vi "sub_DL950_global-settings.vi"(11 "TestType":T1) -> (3 "String":string)   [LabVIEW 2019]
uses:
  Durability/sequence_single.ctl
  _ctrl/rw.ctl
  SubVIs/common/Glob_Ref.vi
  Durability/common/Global 1.vi
panel:
  out "String 2":string
  out "array":string[](array[string])
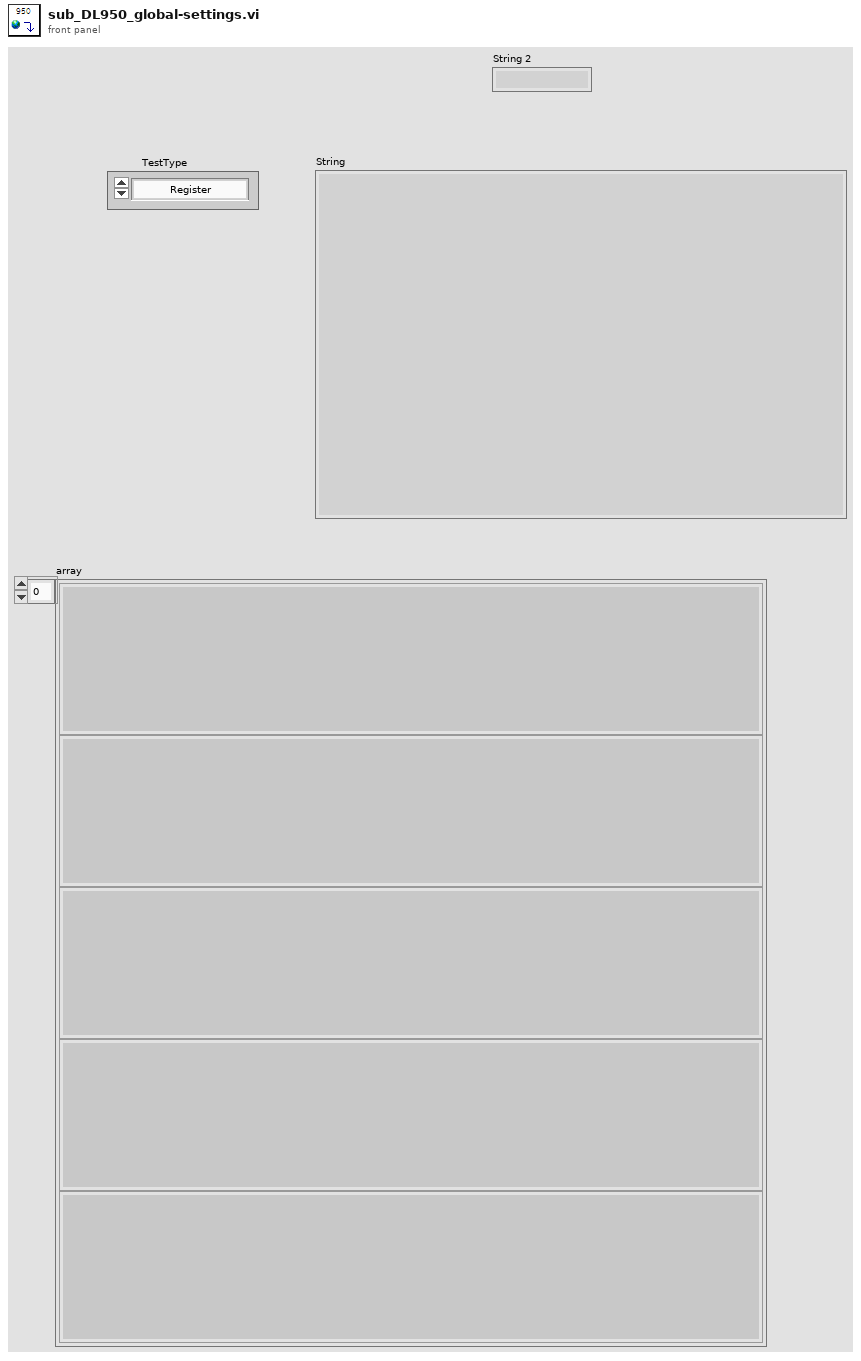
[diagram p1: front panel]
types:
  T1 = typedef "sequence_single.ctl" = enum16{"Register", "RC", "B1", "B2", "B3", "Oper_LV", "Oper_HV", "ContR_LV"}
  T2 = typedef "rw.ctl" = enum16{"read", "write"}
  T3 = typedef "cap_config.ctl" = cluster{"Test Mode":enum32{"6.3.2 저온 작동/방치 시험", "6.3.3 고온 작동/방치 시험", "6.3.4 온도 싸이클 시험", "6.3.6 온습도 싸이클 시험", "6.3.8 결로 시험", "6.3.9 빙결 시험"}, "ON time[ms]":dbl, "OFF time[ms]":dbl, "1. 작동시간[분]":dbl, "2. 미작동시간[분]":dbl, "3. 작동시간[분]":dbl, "level[V]":dbl, "duty":dbl, "Freq":dbl, "Voltage+[V]":dbl, "Voltage-[V]":dbl, "Current+[A]":dbl, "Current-[A]":dbl, "출력전압[V]":dbl, "출력전류[A]":dbl, "OVP Level":dbl, "OCP Level":dbl, "Time Div":u16, "Record Len":i32, "방전 기준[V]":dbl, "Repeate (Each Ch)":u32, "Cycle[N]":u32, "ON/OFF 회 수[N]":dbl, "TrigPos[%]":dbl, "시험시간[분]":dbl}
  T4 = enum32{"6.3.2 저온 작동/방치 시험", "6.3.3 고온 작동/방치 시험", "6.3.4 온도 싸이클 시험", "6.3.6 온습도 싸이클 시험", "6.3.8 결로 시험", "6.3.9 빙결 시험"}
  T5 = cluster{"Freq":dbl, "level[V]":dbl, "duty":dbl, "On time[ms]":dbl}
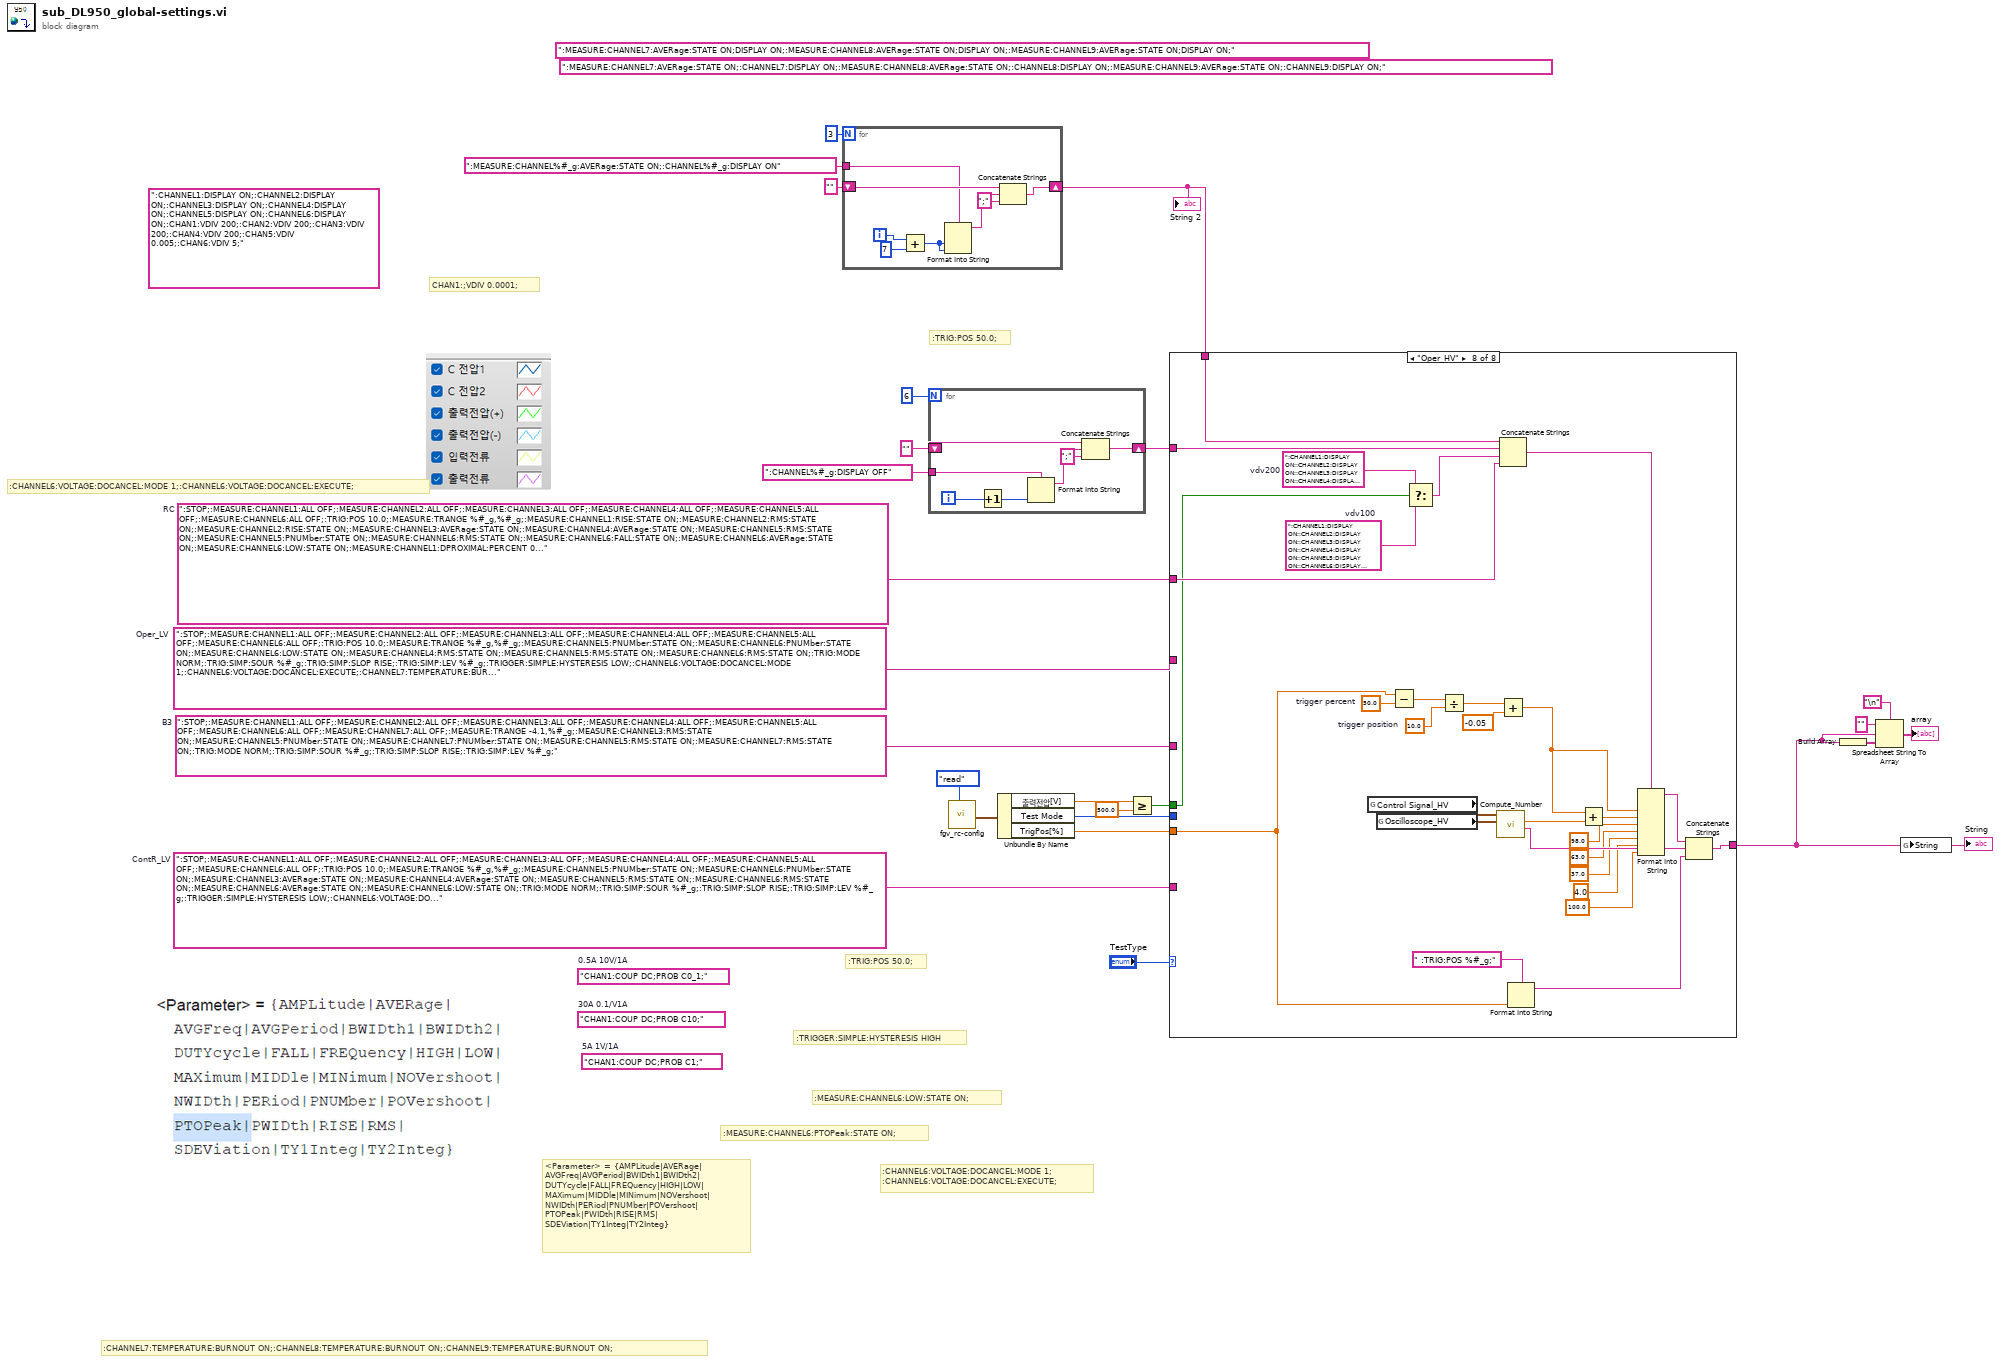
[diagram p0: block diagram]
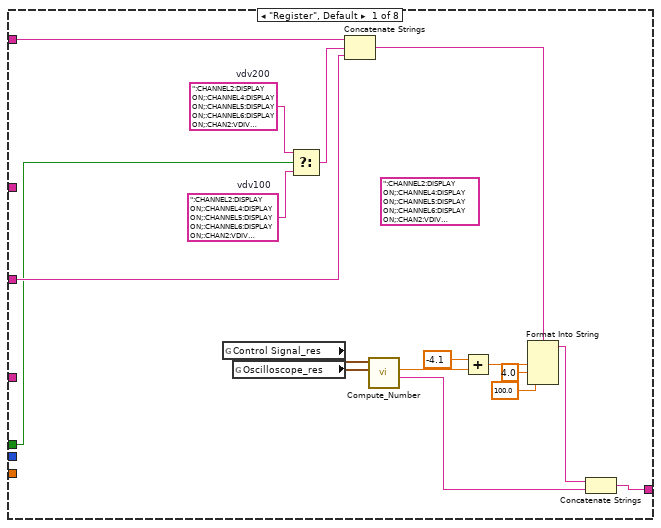
[diagram p2: hidden frame]
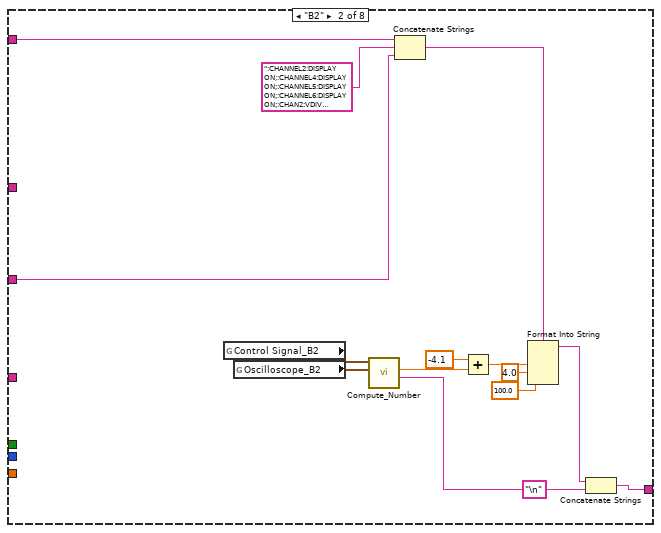
[diagram p3: hidden frame]
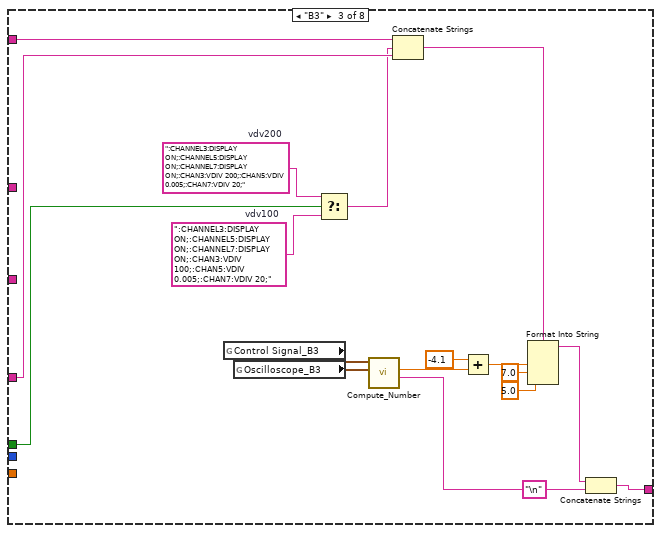
[diagram p4: hidden frame]
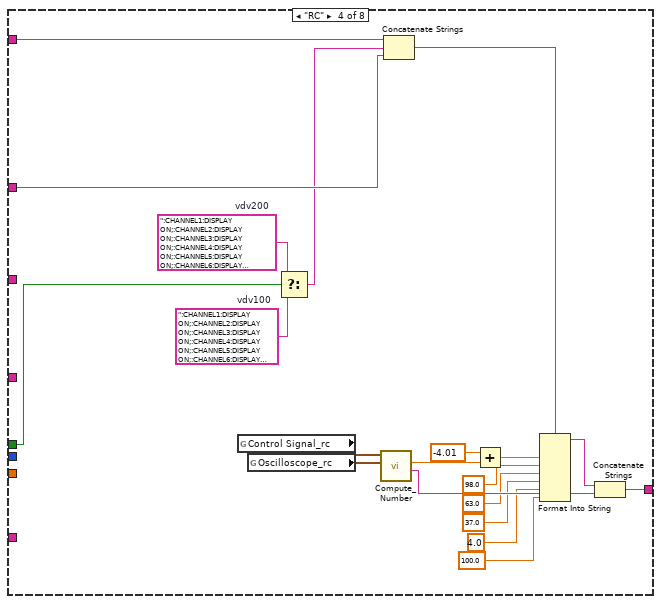
[diagram p5: hidden frame]
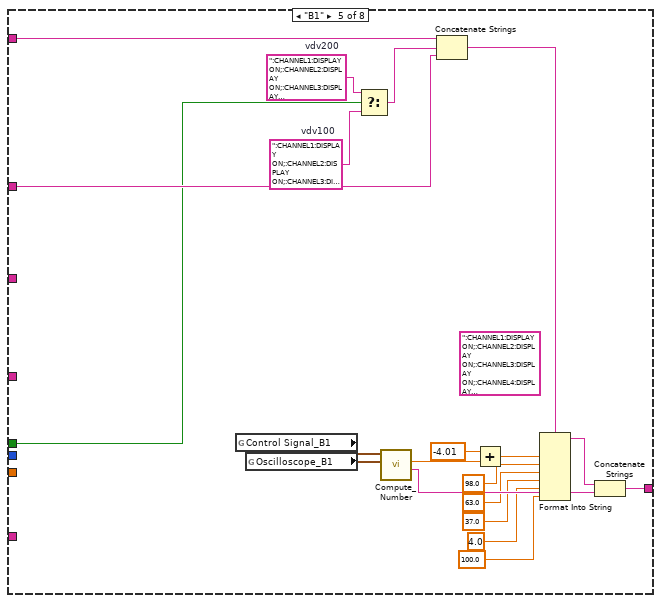
[diagram p6: hidden frame]
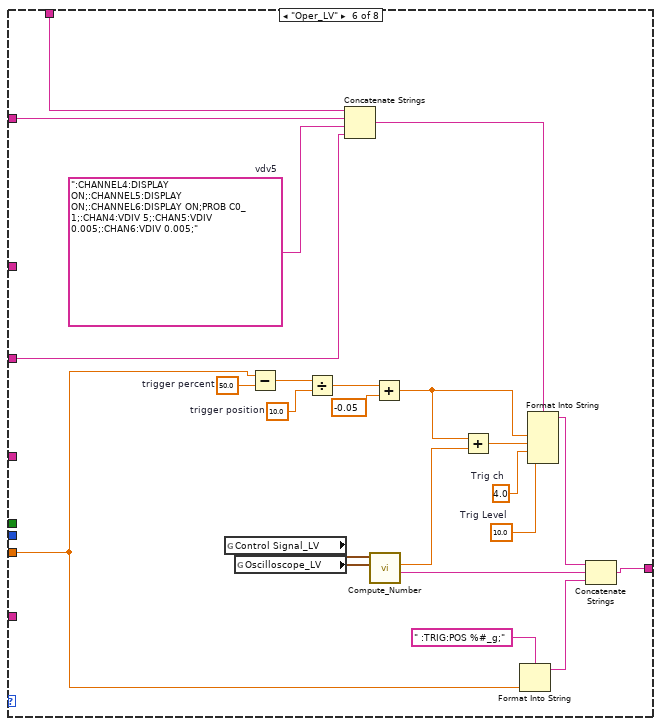
[diagram p7: hidden frame]
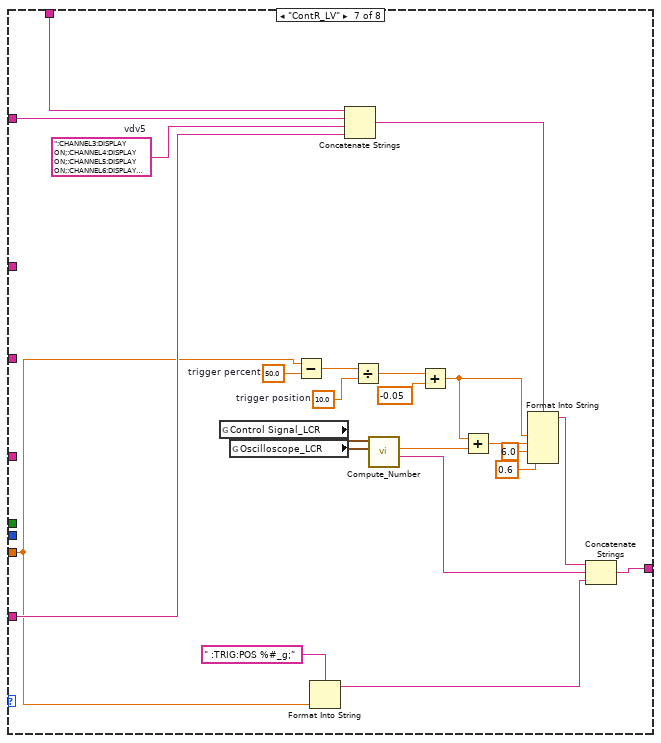
[diagram p8: hidden frame]
diagram:
  (unwired) ":MEASURE:CHANNEL7:AVERage:STATE ON;:CHANNEL7:DISPLAY ON;:MEASURE:CHANNEL8:AVERage:STATE ON;:CHANNEL8:DISPLAY ON;:MEASURE:CHANNEL9:AVERage:STATE ON;:CHANNEL9:DISPLAY ON;" ("String 2")
  (unwired) ":MEASURE:CHANNEL7:AVERage:STATE ON;DISPLAY ON;:MEASURE:CHANNEL8:AVERage:STATE ON;DISPLAY ON;:MEASURE:CHANNEL9:AVERage:STATE ON;DISPLAY ON;" ("String 2")
  (unwired) "CHAN1:COUP DC;PROB C1;"  # 5A 1V/1A
  (unwired) "CHAN1:COUP DC;PROB C10;"  # 30A 0.1/V1A
  (unwired) "CHAN1:COUP DC;PROB C0_1;"  # 0.5A 10V/1A
  w9 = ":STOP;:MEASURE:CHANNEL1:ALL OFF;:MEASURE:CHANNEL2:ALL OFF;:MEASURE:CHANNEL3:ALL OFF;:MEASURE:CHANNEL4:ALL OFF;:MEASURE:CHANNEL5:ALL OFF;:MEASURE:CHANNEL6:ALL OFF;:TRIG:POS 10.0;:MEASURE:TRANGE %#_g,%#_g;:MEASURE:CHANNEL5:PNUMber:STATE ON;:MEASURE:CHANNEL6:PNUMber:STATE ON;:MEASURE:CHANNEL3:AVERage:STATE ON;:MEASURE:CHANNEL4:AVERage:STATE ON;:MEASURE:CHANNEL5:RMS:STATE ON;:MEASURE:CHANNEL6:RMS:STATE ON;:MEASURE:CHANNEL6:AVERage:STATE ON;:MEASURE:CHANNEL6:LOW:STATE ON;:TRIG:MODE NORM;:TRIG:SIMP:SOUR %#_g;:TRIG:SIMP:SLOP RISE;:TRIG:SIMP:LEV %#_g;:TRIGGER:SIMPLE:HYSTERESIS LOW;:CHANNEL6:VOLTAGE:DOCANCEL:MODE 1;:CHANNEL6:VOLTAGE:DOCANCEL:EXECUTE;:CHANNEL7:TEMPERATURE:BURNOUT ON;:CHANNEL8:TEMPERATURE:BURNOUT ON;:CHANNEL9:TEMPERATURE:BURNOUT ON;:CHAN5:BWID 4kHz;"  # ContR_LV
  w10 = ":STOP;:MEASURE:CHANNEL1:ALL OFF;:MEASURE:CHANNEL2:ALL OFF;:MEASURE:CHANNEL3:ALL OFF;:MEASURE:CHANNEL4:ALL OFF;:MEASURE:CHANNEL5:ALL OFF;:MEASURE:CHANNEL6:ALL OFF;:TRIG:POS 10.0;:MEASURE:TRANGE %#_g,%#_g;:MEASURE:CHANNEL5:PNUMber:STATE ON;:MEASURE:CHANNEL6:PNUMber:STATE ON;:MEASURE:CHANNEL6:LOW:STATE ON;:MEASURE:CHANNEL4:RMS:STATE ON;:MEASURE:CHANNEL5:RMS:STATE ON;:MEASURE:CHANNEL6:RMS:STATE ON;:TRIG:MODE NORM;:TRIG:SIMP:SOUR %#_g;:TRIG:SIMP:SLOP RISE;:TRIG:SIMP:LEV %#_g;:TRIGGER:SIMPLE:HYSTERESIS LOW;:CHANNEL6:VOLTAGE:DOCANCEL:MODE 1;:CHANNEL6:VOLTAGE:DOCANCEL:EXECUTE;:CHANNEL7:TEMPERATURE:BURNOUT ON;:CHANNEL8:TEMPERATURE:BURNOUT ON;:CHANNEL9:TEMPERATURE:BURNOUT ON;:CHAN5:BWID 4kHz;"  # Oper_LV
  w16 = ":STOP;:MEASURE:CHANNEL1:ALL OFF;:MEASURE:CHANNEL2:ALL OFF;:MEASURE:CHANNEL3:ALL OFF;:MEASURE:CHANNEL4:ALL OFF;:MEASURE:CHANNEL5:ALL OFF;:MEASURE:CHANNEL6:ALL OFF;:MEASURE:CHANNEL7:ALL OFF;:MEASURE:TRANGE -4.1,%#_g;:MEASURE:CHANNEL3:RMS:STATE ON;:MEASURE:CHANNEL5:PNUMber:STATE ON;:MEASURE:CHANNEL7:PNUMber:STATE ON;:MEASURE:CHANNEL5:RMS:STATE ON;:MEASURE:CHANNEL7:RMS:STATE ON;:TRIG:MODE NORM;:TRIG:SIMP:SOUR %#_g;:TRIG:SIMP:SLOP RISE;:TRIG:SIMP:LEV %#_g;"  # B3
  (unwired) ":CHANNEL1:DISPLAY ON;:CHANNEL2:DISPLAY ON;:CHANNEL3:DISPLAY ON;:CHANNEL4:DISPLAY ON;:CHANNEL5:DISPLAY ON;:CHANNEL6:DISPLAY ON;:CHAN1:VDIV 200;:CHAN2:VDIV 200;:CHAN3:VDIV 200;:CHAN4:VDIV 200;:CHAN5:VDIV 0.005;:CHAN6:VDIV 5;" ("format string")
  w24 = ":STOP;:MEASURE:CHANNEL1:ALL OFF;:MEASURE:CHANNEL2:ALL OFF;:MEASURE:CHANNEL3:ALL OFF;:MEASURE:CHANNEL4:ALL OFF;:MEASURE:CHANNEL5:ALL OFF;:MEASURE:CHANNEL6:ALL OFF;:TRIG:POS 10.0;:MEASURE:TRANGE %#_g,%#_g;:MEASURE:CHANNEL1:RISE:STATE ON;:MEASURE:CHANNEL2:RMS:STATE ON;:MEASURE:CHANNEL2:RISE:STATE ON;:MEASURE:CHANNEL3:AVERage:STATE ON;:MEASURE:CHANNEL4:AVERage:STATE ON;:MEASURE:CHANNEL5:RMS:STATE ON;:MEASURE:CHANNEL5:PNUMber:STATE ON;:MEASURE:CHANNEL6:RMS:STATE ON;:MEASURE:CHANNEL6:FALL:STATE ON;:MEASURE:CHANNEL6:AVERage:STATE ON;:MEASURE:CHANNEL6:LOW:STATE ON;:MEASURE:CHANNEL1:DPROXIMAL:PERCENT 0,30,%#_g;:MEASURE:CHANNEL2:DPROXIMAL:PERCENT 0,30,%#_g;:MEASURE:CHANNEL6:DPROXIMAL:PERCENT %#_g,50,100;:TRIG:MODE NORM;:TRIG:SIMP:SOUR %#_g;:TRIG:SIMP:SLOP RISE;:TRIG:SIMP:LEV %#_g;:TRIGGER:SIMPLE:HYSTERESIS LOW;:CHANNEL7:TEMPERATURE:BURNOUT ON;:CHANNEL8:TEMPERATURE:BURNOUT ON;:CHANNEL9:TEMPERATURE:BURNOUT ON;:CHAN5:BWID 4kHz;:CHANNEL6:VOLTAGE:DOCANCEL:MODE 1;:CHANNEL6:VOLTAGE:DOCANCEL:EXECUTE;"  # RC
  # ":CHANNEL6:VOLTAGE:DOCANCEL:MODE 1;:CHANNEL6:VOLTAGE:DOCANCEL:EXECUTE;"
  # ":CHANNEL7:TEMPERATURE:BURNOUT ON;:CHANNEL8:TEMPERATURE:BURNOUT ON;:CHANNEL9:TEMPERATURE:BURNOUT ON;"
  # ":CHANNEL6:VOLTAGE:DOCANCEL:MODE 1;\n:CHANNEL6:VOLTAGE:DOCANCEL:EXECUTE;"
  # ":MEASURE:CHANNEL6:LOW:STATE ON;"
  # "<Parameter> = {AMPLitude|AVERage|\nAVGFreq|AVGPeriod|BWIDth1|BWIDth2|\nDUTYcycle|FALL|FREQuency|HIGH|LOW|\nMAXimum|MIDDle|MINimum|NOVershoot|\nNWIDth|PERiod|PNUMber|POVershoot|\nPTOPeak|PWIDth|RISE|RMS|\nSDEViation|TY1Integ|TY2Integ}"
  # ":MEASURE:CHANNEL6:PTOPeak:STATE ON;"
  # ":TRIG:POS 50.0;"
  # ":TRIGGER:SIMPLE:HYSTERESIS HIGH"
  # ":TRIG:POS 50.0;"
  # "CHAN1:;VDIV 0.0001;"
  n1 = for {
    N: 3 -> [_]
    shift-right: [w32] -> w5
    shift-left: "" -> [w31]
    tunnel: ":MEASURE:CHANNEL%#_g:AVERage:STATE ON;:CHANNEL%#_g:DISPLAY ON" ("format string") -> [w27]
    i -> [w29]
    n2 = Add(x=w29, y=7) -> (x+y=w26:i32)
    n3 = Format Into String(format string=w27, w26, w26) -> (resulting string=w33:string)  [unwired: 2 in, 1 out]
    n4 = Concatenate Strings(w31, w33, ";" ("string")) -> (w32:string)
  }
  "String 2" <- w5
  n5 = for {
    N: 6 -> [_]
    shift-right: [w37] -> w17
    shift-left: "" -> [w36]
    tunnel: ":CHANNEL%#_g:DISPLAY OFF" ("format string") -> [w34]
    i -> [w40]
    n6 = Increment(x=w40) -> (x+1=w39:i32)
    n7 = Format Into String(format string=w34, w39) -> (resulting string=w38:string)  [unwired: 2 in, 1 out]
    n8 = Concatenate Strings(w36, w38, ";" ("string")) -> (w37:string)
  }
  n9 = call "fgv_rc-config.vi"("cmd"=rw."read") -> ("Testconfig out"=w14:T3)  [unwired: 9 in, 1 out]
  n10 = Unbundle By Name(w14) -> ("출력전압[V]"=w13:dbl, "Test Mode"=w4:T4, "TrigPos[%]"=w2:dbl)
  n11 = Greater Or Equal?(x=w13, y=500.0) -> (x >= y?=w11:bool)
  n12 = case shown="\"Oper_HV\"" "TestType" {
    tunnel: [w52 w64 w81 w102 w122 w151 w171 w198] -> w3
    tunnel: w24 -> [_ _ _ w94 w115 _ _ w190]
    tunnel: w10 -> [w46 w59 _ _ _ w149 _ _]
    tunnel: w17 -> [w47 w60 w78 w95 w114 w150 w166 w191]
    tunnel: w16 -> [_ _ w76 _ _ _ _ _]
    tunnel: w11 -> [w42 _ w75 w92 w109 _ _ w188]
    tunnel: w9 -> [_ _ _ _ _ _ w163 _]
    tunnel: w5 -> [_ _ _ _ _ w148 w161 w184]
    tunnel: w4 -> [_ _ _ _ _ _ _ _]
    tunnel: w2 -> [_ _ _ _ _ w147 w153 w176]
    frame "Register", Default {
      w44 = ":CHANNEL2:DISPLAY ON;:CHANNEL4:DISPLAY ON;:CHANNEL5:DISPLAY ON;:CHANNEL6:DISPLAY ON;:CHAN2:VDIV 100;:CHAN4:VDIV 100;:CHAN5:VDIV 0.005;:CHAN6:VDIV 5;"  # vdv100
      w43 = ":CHANNEL2:DISPLAY ON;:CHANNEL4:DISPLAY ON;:CHANNEL5:DISPLAY ON;:CHANNEL6:DISPLAY ON;:CHAN2:VDIV 200;:CHAN4:VDIV 200;:CHAN5:VDIV 0.005;:CHAN6:VDIV 5;"  # vdv200
      (unwired) ":CHANNEL2:DISPLAY ON;:CHANNEL4:DISPLAY ON;:CHANNEL5:DISPLAY ON;:CHANNEL6:DISPLAY ON;:CHAN2:VDIV 200;:CHAN4:VDIV 200;:CHAN5:VDIV 0.005;:CHAN6:VDIV 5;" ("format string")
      n13 = global read "Glob_Ref.vi" "Control Signal_res"() -> (w54:T5)
      n14 = global read "Glob_Ref.vi" "Oscilloscope_res"() -> (w55:cluster{"Record Len":i32, "Time Div":u16})
      n15 = Select(t=w43, s=w42, f=w44) -> (s? t:f=w41:string)
      n16 = Concatenate Strings(w47, w41, w46) -> (w45:string)
      n17 = call "Compute_Number.vi"("Oscilloscope"=w55, "Control Signal"=w54) -> ("output string"=w51:string, "NumDiv"=w56:dbl)  [unwired: 6 in, 2 out]
      n18 = Add(x=-4.1, y=w56) -> (x+y=w57:dbl)
      n19 = Format Into String(format string=w45, w57, 4.0 ("input 2"), 100.0 ("input 3")) -> (resulting string=w48:string)  [unwired: 2 in, 1 out]
      n20 = Concatenate Strings(w48, w51) -> (w52:string)
    }
    frame "B2" {
      (unwired) "\n" ("string")
      n21 = global read "Glob_Ref.vi" "Control Signal_B2"() -> (w68:T5)
      n22 = global read "Glob_Ref.vi" "Oscilloscope_B2"() -> (w69:cluster{"Record Len":i32, "Time Div":u16})
      n23 = call "Compute_Number.vi"("Oscilloscope"=w69, "Control Signal"=w68) -> ("output string"=w65:string, "NumDiv"=w70:dbl)  [unwired: 6 in, 2 out]
      n24 = Concatenate Strings(w60, ":CHANNEL2:DISPLAY ON;:CHANNEL4:DISPLAY ON;:CHANNEL5:DISPLAY ON;:CHANNEL6:DISPLAY ON;:CHAN2:VDIV 200;:CHAN4:VDIV 200;:CHAN5:VDIV 0.005;:CHAN6:VDIV 5;" ("format string"), w59) -> (w58:string)
      n25 = Add(x=-4.1, y=w70) -> (x+y=w71:dbl)
      n26 = Format Into String(format string=w58, w71, 4.0 ("input 2"), 100.0 ("input 3")) -> (resulting string=w66:string)  [unwired: 2 in, 1 out]
      n27 = Concatenate Strings(w66, w65) -> (w64:string)
    }
    frame "B3" {
      w73 = ":CHANNEL3:DISPLAY ON;:CHANNEL5:DISPLAY ON;:CHANNEL7:DISPLAY ON;:CHAN3:VDIV 100;:CHAN5:VDIV 0.005;:CHAN7:VDIV 20;"  # vdv100
      w74 = ":CHANNEL3:DISPLAY ON;:CHANNEL5:DISPLAY ON;:CHANNEL7:DISPLAY ON;:CHAN3:VDIV 200;:CHAN5:VDIV 0.005;:CHAN7:VDIV 20;"  # vdv200
      (unwired) "\n" ("string")
      n28 = global read "Glob_Ref.vi" "Control Signal_B3"() -> (w85:T5)
      n29 = global read "Glob_Ref.vi" "Oscilloscope_B3"() -> (w86:cluster{"Record Len":i32, "Time Div":u16})
      n30 = Select(t=w74, s=w75, f=w73) -> (s? t:f=w72:string)
      n31 = call "Compute_Number.vi"("Oscilloscope"=w86, "Control Signal"=w85) -> ("output string"=w82:string, "NumDiv"=w87:dbl)  [unwired: 6 in, 2 out]
      n32 = Concatenate Strings(w78, w72, w76) -> (w77:string)
      n33 = Add(x=-4.1, y=w87) -> (x+y=w88:dbl)
      n34 = Format Into String(format string=w77, w88, 7.0 ("input 2"), 5.0 ("input 3")) -> (resulting string=w83:string)  [unwired: 2 in, 1 out]
      n35 = Concatenate Strings(w83, w82) -> (w81:string)
    }
    frame "RC" {
      w90 = ":CHANNEL1:DISPLAY ON;:CHANNEL2:DISPLAY ON;:CHANNEL3:DISPLAY ON;:CHANNEL4:DISPLAY ON;:CHANNEL5:DISPLAY ON;:CHANNEL6:DISPLAY ON;:CHAN1:VDIV 200;:CHAN2:VDIV 200;:CHAN3:VDIV 200;:CHAN4:VDIV 200;:CHAN5:VDIV 0.005;:CHAN6:VDIV 5;"  # vdv200
      w91 = ":CHANNEL1:DISPLAY ON;:CHANNEL2:DISPLAY ON;:CHANNEL3:DISPLAY ON;:CHANNEL4:DISPLAY ON;:CHANNEL5:DISPLAY ON;:CHANNEL6:DISPLAY ON;:CHAN1:VDIV 100;:CHAN2:VDIV 100;:CHAN3:VDIV 100;:CHAN4:VDIV 100;:CHAN5:VDIV 0.005;:CHAN6:VDIV 5;"  # vdv100
      n36 = global read "Glob_Ref.vi" "Control Signal_rc"() -> (w107:T5)
      n37 = global read "Glob_Ref.vi" "Oscilloscope_rc"() -> (w106:cluster{"Record Len":i32, "Time Div":u16})
      n38 = Select(t=w90, s=w92, f=w91) -> (s? t:f=w89:string)
      n39 = call "Compute_Number.vi"("Oscilloscope"=w106, "Control Signal"=w107) -> ("output string"=w101:string, "NumDiv"=w105:dbl)  [unwired: 6 in, 2 out]
      n40 = Concatenate Strings(w95, w89, w94) -> (w93:string)
      n41 = Add(x=-4.01, y=w105) -> (x+y=w104:dbl)
      n42 = Format Into String(format string=w93, w104, 98.0 ("input 2"), 63.0 ("input 3"), 37.0 ("input 4"), 4.0 ("input 4"), 100.0 ("input 4")) -> (resulting string=w108:string)  [unwired: 2 in, 1 out]
      n43 = Concatenate Strings(w108, w101) -> (w102:string)
    }
    frame "B1" {
      w112 = ":CHANNEL1:DISPLAY ON;:CHANNEL2:DISPLAY ON;:CHANNEL3:DISPLAY ON;:CHANNEL4:DISPLAY ON;:CHANNEL5:DISPLAY ON;:CHANNEL6:DISPLAY ON;:CHAN1:VDIV 100;:CHAN2:VDIV 100;:CHAN3:VDIV 100;:CHAN4:VDIV 100;:CHAN5:VDIV 0.005;:CHAN6:VDIV 5;"  # vdv100
      w111 = ":CHANNEL1:DISPLAY ON;:CHANNEL2:DISPLAY ON;:CHANNEL3:DISPLAY ON;:CHANNEL4:DISPLAY ON;:CHANNEL5:DISPLAY ON;:CHANNEL6:DISPLAY ON;:CHAN1:VDIV 200;:CHAN2:VDIV 200;:CHAN3:VDIV 200;:CHAN4:VDIV 200;:CHAN5:VDIV 0.005;:CHAN6:VDIV 5;"  # vdv200
      (unwired) ":CHANNEL1:DISPLAY ON;:CHANNEL2:DISPLAY ON;:CHANNEL3:DISPLAY ON;:CHANNEL4:DISPLAY ON;:CHANNEL5:DISPLAY ON;:CHANNEL6:DISPLAY ON;:CHAN1:VDIV 200;:CHAN2:VDIV 200;:CHAN3:VDIV 200;:CHAN4:VDIV 200;:CHAN5:VDIV 0.005;:CHAN6:VDIV 5;" ("format string")
      n44 = global read "Glob_Ref.vi" "Control Signal_B1"() -> (w127:T5)
      n45 = global read "Glob_Ref.vi" "Oscilloscope_B1"() -> (w126:cluster{"Record Len":i32, "Time Div":u16})
      n46 = Select(t=w111, s=w109, f=w112) -> (s? t:f=w110:string)
      n47 = call "Compute_Number.vi"("Oscilloscope"=w126, "Control Signal"=w127) -> ("output string"=w121:string, "NumDiv"=w125:dbl)  [unwired: 6 in, 2 out]
      n48 = Concatenate Strings(w114, w110, w115) -> (w113:string)
      n49 = Add(x=-4.01, y=w125) -> (x+y=w124:dbl)
      n50 = Format Into String(format string=w113, w124, 98.0 ("input 2"), 63.0 ("input 3"), 37.0 ("input 4"), 4.0 ("input 4"), 100.0 ("input 4")) -> (resulting string=w128:string)  [unwired: 2 in, 1 out]
      n51 = Concatenate Strings(w128, w121) -> (w122:string)
    }
    frame "Oper_LV" {
      w135 = 10.0  # trigger position
      w134 = 50.0  # trigger percent
      w137 = ":CHANNEL4:DISPLAY ON;:CHANNEL5:DISPLAY ON;:CHANNEL6:DISPLAY ON;PROB C0_1;:CHAN4:VDIV 5;:CHAN5:VDIV 0.005;:CHAN6:VDIV 0.005;"  # vdv5
      w140 = 10.0  # Trig Level
      w141 = 4.0  # Trig ch
      n52 = global read "Glob_Ref.vi" "Control Signal_LV"() -> (w143:T5)
      n53 = global read "Glob_Ref.vi" "Oscilloscope_LV"() -> (w144:cluster{"Record Len":i32, "Time Div":u16})
      n54 = Subtract(x=w147, y=w134) -> (x-y=w136:dbl)
      n55 = Divide(x=w136, y=w135) -> (x/y=w133:dbl)
      n56 = Concatenate Strings(w148, w150, w137, w149) -> (w138:string)
      n57 = call "Compute_Number.vi"("Oscilloscope"=w144, "Control Signal"=w143) -> ("output string"=w142:string, "NumDiv"=w145:dbl)  [unwired: 6 in, 2 out]
      n58 = Add(x=w133, y=-0.05) -> (x+y=w131:dbl)
      n59 = Add(x=w131, y=w145) -> (x+y=w146:dbl)
      n60 = Format Into String(format string=" :TRIG:POS %#_g;", w147) -> (resulting string=w129:string)  [unwired: 2 in, 1 out]
      n61 = Format Into String(format string=w138, w131, w146, w141, w140) -> (resulting string=w139:string)  [unwired: 2 in, 1 out]
      n62 = Concatenate Strings(w139, w142, w129) -> (w151:string)
    }
    frame "ContR_LV" {
      w159 = 10.0  # trigger position
      w158 = 50.0  # trigger percent
      w164 = ":CHANNEL3:DISPLAY ON;:CHANNEL4:DISPLAY ON;:CHANNEL5:DISPLAY ON;:CHANNEL6:DISPLAY ON;PROB C1;:CHAN3:VDIV 5;:CHAN4:VDIV 5;:CHAN5:VDIV 0.005;:CHAN6:VDIV 0.5;"  # vdv5
      n63 = global read "Glob_Ref.vi" "Control Signal_LCR"() -> (w172:T5)
      n64 = global read "Glob_Ref.vi" "Oscilloscope_LCR"() -> (w173:cluster{"Record Len":i32, "Time Div":u16})
      n65 = Subtract(x=w153, y=w158) -> (x-y=w160:dbl)
      n66 = Format Into String(format string=" :TRIG:POS %#_g;", w153) -> (resulting string=w152:string)  [unwired: 2 in, 1 out]
      n67 = Concatenate Strings(w161, w166, w164, w163) -> (w165:string)
      n68 = Divide(x=w160, y=w159) -> (x/y=w157:dbl)
      n69 = call "Compute_Number.vi"("Oscilloscope"=w173, "Control Signal"=w172) -> ("output string"=w170:string, "NumDiv"=w162:dbl)  [unwired: 6 in, 2 out]
      n70 = Add(x=w157, y=-0.05) -> (x+y=w155:dbl)
      n71 = Add(x=w155, y=w162) -> (x+y=w174:dbl)
      n72 = Format Into String(format string=w165, w155, w174, 6.0 ("input 2"), 0.6 ("input 3")) -> (resulting string=w167:string)  [unwired: 2 in, 1 out]
      n73 = Concatenate Strings(w167, w170, w152) -> (w171:string)
    }
    frame "Oper_HV" {
      w182 = 10.0  # trigger position
      w181 = 50.0  # trigger percent
      w186 = ":CHANNEL1:DISPLAY ON;:CHANNEL2:DISPLAY ON;:CHANNEL3:DISPLAY ON;:CHANNEL4:DISPLAY ON;:CHANNEL5:DISPLAY ON;:CHANNEL6:DISPLAY ON;:CHAN1:VDIV 200;:CHAN2:VDIV 200;:CHAN3:VDIV 200;:CHAN4:VDIV 200;:CHAN5:VDIV 0.005;:CHAN6:VDIV 5;PROB C10;"  # vdv200
      w187 = ":CHANNEL1:DISPLAY ON;:CHANNEL2:DISPLAY ON;:CHANNEL3:DISPLAY ON;:CHANNEL4:DISPLAY ON;:CHANNEL5:DISPLAY ON;:CHANNEL6:DISPLAY ON;:CHAN1:VDIV 100;:CHAN2:VDIV 100;:CHAN3:VDIV 100;:CHAN4:VDIV 100;:CHAN5:VDIV 0.005;:CHAN6:VDIV 5;PROB C10;"  # vdv100
      n74 = global read "Glob_Ref.vi" "Control Signal_HV"() -> (w202:T5)
      n75 = global read "Glob_Ref.vi" "Oscilloscope_HV"() -> (w201:cluster{"Record Len":i32, "Time Div":u16})
      n76 = Subtract(x=w176, y=w181) -> (x-y=w183:dbl)
      n77 = Select(t=w186, s=w188, f=w187) -> (s? t:f=w185:string)
      n78 = Divide(x=w183, y=w182) -> (x/y=w180:dbl)
      n79 = call "Compute_Number.vi"("Oscilloscope"=w201, "Control Signal"=w202) -> ("output string"=w197:string, "NumDiv"=w200:dbl)  [unwired: 6 in, 2 out]
      n80 = Concatenate Strings(w184, w191, w185, w190) -> (w189:string)
      n81 = Add(x=w180, y=-0.05) -> (x+y=w178:dbl)
      n82 = Format Into String(format string=" :TRIG:POS %#_g;", w176) -> (resulting string=w175:string)  [unwired: 2 in, 1 out]
      n83 = Add(x=w178, y=w200) -> (x+y=w199:dbl)
      n84 = Format Into String(format string=w189, w178, w199, 98.0 ("input 2"), 63.0 ("input 3"), 37.0 ("input 4"), 4.0 ("input 4"), 100.0 ("input 4")) -> (resulting string=w203:string)  [unwired: 2 in, 1 out]
      n85 = Concatenate Strings(w203, w197, w175) -> (w198:string)
    }
  }
  "String" <- w3
  n86 = Build Array(w3) -> (w23:string[])
  n87 = Spreadsheet String To Array(delimiter (Tab)="\n", format string="", spreadsheet string=w3, array type (2D Dbl)=w23) -> (array=→"array":string[])
  n88 = global write "Global 1.vi" "String"(w3) -> ()
